vi "Configure External Trigger.vi"(5 "Enable External Trigger Delay (T:Enable)":bool=TRUE, 6 "External Trigger Slope (0: Negative)":u16(ring) items=["Negative", "Positive"], 7 "External Trigger Delay (0 bit)":dbl, 8 "error in (no error)":errorcluster, 9 "External Trigger Source (0: Pattern Trigger Input1)":u16(ring) items=["Pattern Trigger Input1", "Pattern Trigger Input2"], 10 "Modulation Format (0: Custom)":u16(ring) items=["Custom", "Dual Modulation", "Dual ARB"], 11 "VISA resource name":refnum<visa-resource-name>) -> (0 "error out":errorcluster, 3 "VISA resource name out":refnum<visa-resource-name>)   [LabVIEW 2009, in "Agilent PSG MXG Series.lvlib"]
doc: "Configures the external trigger source, trigger delay and polarity for the specific modulation format.\n\n<B>Notes:</B>\n(1) This VI is valid only in E8267C, E8267D, N5182A.\n\n(2) For E8267C, this VI is valid only when the instrument installs <B>Option 002</B> (Internal baseband generator) or <B>Option 602</B> (Digital bus baseband generator).\n\n(3) For E8267D, this VI is valid only when the instrument installs <B>Option 601</B> or <B>Option 602</B> (Internal baseband generator).\n\n(4) For N5182A, this VI is valid only when the instrument installs <B>Option 651</B> or <B>Option 652</B> or <B>Option 654</B> (Internal baseband generator)."
uses:
  Agilent PSG MXG Series.lvlib
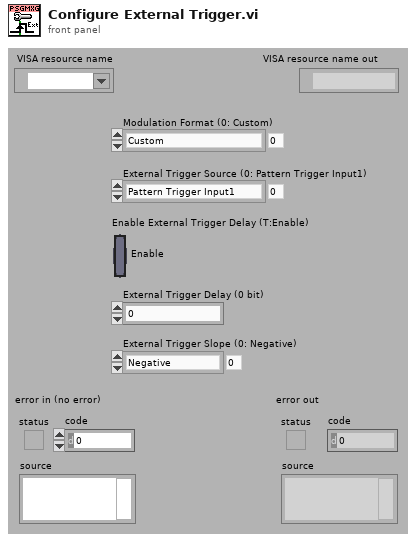
[diagram p1: front panel]
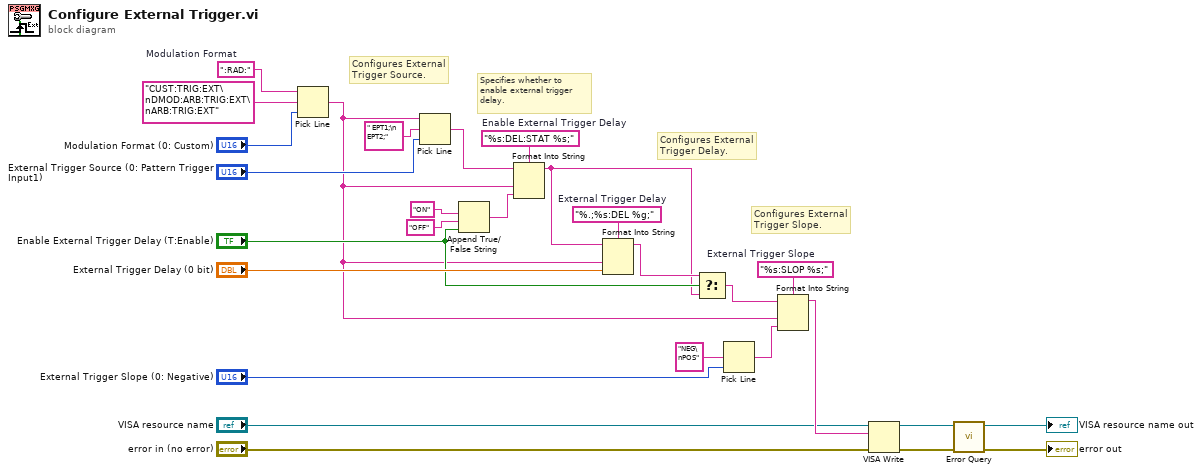
[diagram p0: block diagram]
diagram:
  w13 = "%s:SLOP %s;"  # External Trigger Slope
  w18 = "%.;%s:DEL %g;"  # External Trigger Delay
  w23 = "%s:DEL:STAT %s;"  # Enable External Trigger Delay
  w28 = ":RAD:"  # Modulation Format
  # "Configures External\nTrigger Slope."
  # "Configures External\nTrigger Delay."
  # "Specifies whether to\nenable external trigger\ndelay."
  # "Configures External\nTrigger Source."
  n1 = Pick Line(string ("")=w28, multi-line string="CUST:TRIG:EXT\nDMOD:ARB:TRIG:EXT\nARB:TRIG:EXT", line index="Modulation Format (0: Custom)") -> (output string=w11:string)
  n2 = Pick Line(string ("")=w11, multi-line string=" EPT1;\n EPT2;", line index="External Trigger Source (0: Pattern Trigger Input1)") -> (output string=w22:string)
  n3 = Append True/False String(1:"Enable External Trigger Delay (T:Enable)", 2:"OFF" ("false string"), 3:"ON" ("true string")) -> (0:w21:string)  [unwired: 1 out]
  n4 = Format Into String(format string=w23, initial string=w22, w11, w21) -> (resulting string=w14:string)  [unwired: 1 in, 1 out]
  n5 = Format Into String(format string=w18, initial string=w14, w11, "External Trigger Delay (0 bit)") -> (resulting string=w15:string)  [unwired: 1 in, 1 out]
  n6 = Select(t=w15, s="Enable External Trigger Delay (T:Enable)", f=w14) -> (s? t:f=w12:string)
  n7 = Pick Line(multi-line string="NEG\nPOS", line index="External Trigger Slope (0: Negative)") -> (output string=w10:string)  [unwired: 1 out]
  n8 = Format Into String(format string=w13, initial string=w12, w11, w10) -> (resulting string=w7:string)  [unwired: 1 in, 1 out]
  n9 = VISA Write(VISA resource name="VISA resource name", write buffer=w7, error in (no error)="error in (no error)") -> (VISA resource name out=w6:refnum<visa-resource-name>, error out=w5:errorcluster)  [unwired: 1 out]
  n10 = call "Error Query.vi"("error in (no error)"=w5, "VISA resource name"=w6) -> ("error out"=→"error out":errorcluster, "VISA resource name out"=→"VISA resource name out":refnum<visa-resource-name>)  [unwired: 8 out]
